vi "FindFirstTouch.vi"(6 "EN":bool, 8 "Level Reference":dbl, 11 "Analog FW In":T1) -> (1 "CounterDeleteOut":i32, 2 "TotalSizeOut":i32, 3 "Analog FW Out":T1)   [LabVIEW 2017]
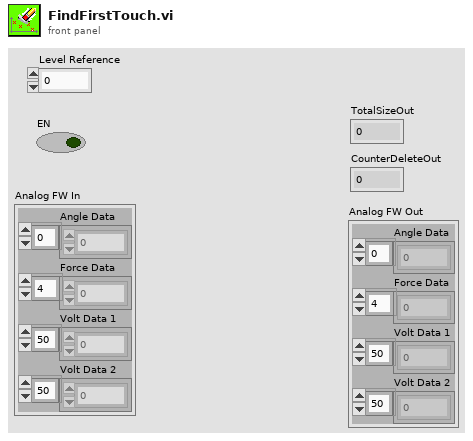
[diagram p1: front panel]
types:
  T1 = cluster{"Angle Data":dbl[], "Force Data":dbl[], "Volt Data 1":dbl[], "Volt Data 2":dbl[]}
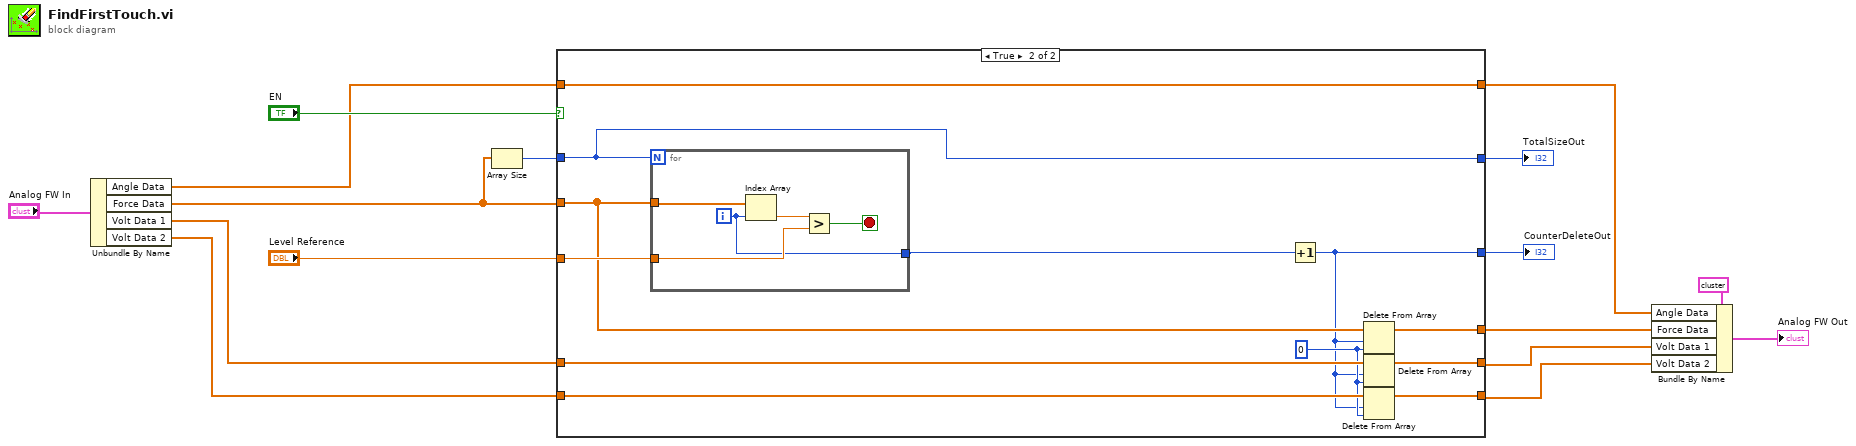
[diagram p0: block diagram]
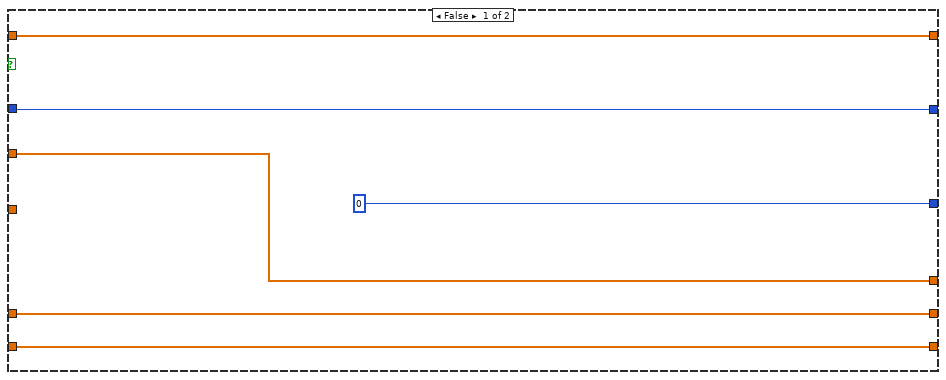
[diagram p2: hidden frame]
diagram:
  n1 = Unbundle By Name("Analog FW In") -> ("Angle Data"=w1:dbl[], "Force Data"=w5:dbl[], "Volt Data 1"=w10:dbl[], "Volt Data 2"=w9:dbl[])
  n2 = Array Size(array=w5) -> (size(s)=w4:i32)
  n3 = case shown="True" "EN" {
    tunnel: "Level Reference" -> [_ w34]
    tunnel: w5 -> [w22 w33]
    tunnel: [w22 w32] -> w11
    tunnel: w10 -> [w21 w31]
    tunnel: w9 -> [w20 w30]
    tunnel: [w21 w28] -> w8
    tunnel: [w20 w27] -> w7
    tunnel: [0 w26] -> w6
    tunnel: w4 -> [w19 w25]
    tunnel: [w19 w25] -> w3
    tunnel: [w17 w24] -> w2
    tunnel: w1 -> [w17 w24]
    frame False {
    }
    frame True {
      w29 = 0 ("index")
      n4 = for {
        N: w25 -> [_]
        tunnel: w33 -> [w39]
        tunnel: w34 -> [w37]
        tunnel: [w35] -> w23
        i -> [w35]
        stop <- w36 stop-if-true
        n5 = Index Array(array=w39, index=w35) -> (element=w38:dbl)
        n6 = Greater?(x=w38, y=w37) -> (0:w36:bool)
      }
      n7 = Increment(x=w23) -> (x+1=w26:i32)
      n8 = Delete From Array "Delete From Array"(array=w33, length=w26, index=w29) -> (array with subset deleted=w32:dbl[])  [unwired: 1 out]
      n9 = Delete From Array(array=w31, length=w26, index=w29) -> (array with subset deleted=w28:dbl[])  [unwired: 1 out]
      n10 = Delete From Array(array=w30, length=w26, index=w29) -> (array with subset deleted=w27:dbl[])  [unwired: 1 out]
    }
  }
  "CounterDeleteOut" <- w6
  "TotalSizeOut" <- w3
  n11 = Bundle By Name(cluster=T1 {"Angle Data"=[], "Force Data"=[0.0, 0.035, 0.005, 0.035, 0.035, 0.035, 0.035, 0.005, 0.005, 0.035, 0.035, 0.035, 0.035, 0.005, 0.065, 0.035, 0.005, 0.035, 0.005, 0.005, 0.005, 0.005, 0.065, 0.035, 0.035, 0.005, 0.035, 0.035, 0.035, 0.065, 0.035, 0.065, 0.035, 0.035, 0.035, 0.035, 0.005, 0.065, 0.035, 0.005, 0.035, 0.035, 0.005, 0.005, 0.035, 0.035, 0.005, 0.065, 0.005, 0.035, 0.026, 0.035, 0.005, 0.035, 0.065, 0.035, 0.035, 0.005, 0.005, 0.035, 0.035, 0.005, 0.005, 0.065, 0.035, 0.035, 0.035, 0.005, 0.065, 0.005, 0.035, 0.005, 0.065, 0.096, 0.065, 0.065, 0.096, 0.035, 0.065, 0.065, 0.096, 0.096, 0.096, 0.096, 0.126, 0.096, 0.096, 0.126, 0.096, 0.126, 0.126, 0.096, 0.218, 0.157, 0.157, 0.187, 0.157, 0.157, 0.187, 0.157, 0.187, 0.218, 0.187, 0.187, 0.187, 0.218, 0.218, 0.248, 0.279, 0.279, 0.279, 0.34, 0.279, 0.279, 0.279, 0.309, 0.279, 0.279, 0.309, 0.34, 0.37, 0.309, 0.37, 0.34, 0.34, 0.401, 0.401, 0.37, 0.401, 0.401, 0.401, 0.37, 0.431, 0.431, 0.431, 0.431, 0.401, 0.462, 0.401, 0.431, 0.431, 0.431, 0.462, 0.431, 0.431, 0.431, 0.431, 0.462, 0.431, 0.431, 0.462, 0.431, 0.431, 0.431, 0.462, 0.431, 0.431, 0.462, 0.401, 0.462, 0.431, 0.431, 0.431, 0.431, 0.462, 0.462, 0.431, 0.462, 0.431, 0.492, 0.431, 0.462, 0.492, 0.431, 0.492, 0.492, 0.492, 0.431, 0.431, 0.522, 0.492, 0.431, 0.462, 0.462, 0.462, 0.492, 0.431, 0.431, 0.431, 0.431, 0.462, 0.462, 0.462, 0.462, 0.401, 0.492, 0.431, 0.431, 0.431, 0.431, 0.431, 0.431, 0.431, 0.431, 0.462, 0.401, 0.431, 0.431, 0.431, 0.431, 0.401, 0.431, 0.431, 0.431, 0.37, 0.431, 0.401, 0.431, 0.401, 0.431, 0.401, 0.431, 0.431, 0.522, 0.462, 0.492, 0.492, 0.522, 0.462, 0.522, 0.522, 0.553, 0.553, 0.553, 0.583, 0.553, 0.583, 0.553, 0.553, 0.553, 0.583, 0.583, 0.614, 0.644, 0.614, 0.614, 0.644, 0.644, 0.644, 0.675, 0.644, 0.675, 0.644, 0.675, 0.705, 0.644, 0.705, 0.766, 0.736, 0.736, 0.766, 0.736, 0.766, 0.766, 0.736, 0.797, 0.766, 0.797, 0.797, 0.766, 0.766, 0.766, 0.797, 0.766, 0.827, 0.827, 0.827, 0.797, 0.827, 0.827, 0.858, 0.858, 0.827, 0.827, 0.766, 0.675, 0.583, 0.492, 0.492, 0.492, 0.492, 0.492, 0.492, 0.492, 0.492, 0.431, 0.462, 0.401, 0.462, 0.462, 0.431, 0.462, 0.462, 0.431, 0.462, 0.462, 0.431, 0.462, 0.462, 0.431, 0.431, 0.462, 0.401, 0.401, 0.431, 0.431, 0.431, 0.431, 0.431, 0.401, 0.431, 0.431, 0.401, 0.431, 0.431, 0.431, 0.431, 0.431, 0.431, 0.431, 0.462, 0.431, 0.462, 0.431, 0.401, 0.431, 0.462, 0.431, 0.492, 0.431, 0.522, 0.553, 0.614, 0.644, 0.644, 0.705, 0.736, 0.797, 0.827, 0.858, 0.888, 0.919, 0.919, 0.949, 1.01, 1.01, 1.04, 1.04, 1.132, 1.101, 1.132, 1.132, 1.162, 1.193, 1.223, 1.254, 1.254, 1.284, 1.315, 1.315, 1.376, 1.436, 1.376, 1.467, 1.467, 1.497, 1.497, 1.589, 1.558, 1.589, 1.619, 1.65, 1.68, 1.741, 1.711, 1.802, 1.802, 1.833, 1.863, 1.893, 1.924, 1.954, 1.985, 1.954, 1.954, 1.954, 1.954, 1.924, 1.924, 1.924, 1.954, 1.924, 1.924, 1.893, 1.954, 1.863, 1.893, 1.893, 1.863, 1.893, 1.893, 1.893, 1.893, 1.893, 1.924, 1.893, 1.924, 1.863, 1.863, 1.863, 1.893, 1.893, 1.863, 1.863, 1.893, 1.863, 1.863, 1.863, 1.893, 1.893, 1.833, 1.893, 1.863, 1.863, 1.802, 1.863, 1.833, 1.863, 1.863], "Volt Data 1"=array[439 elements], "Volt Data 2"=[0.0, 0.036, 0.036, 0.066, 0.005, 0.025, 0.036, 0.036, 0.025, 0.117, 0.036, 0.025, 0.056, 0.066, 0.056, 0.086, 0.036, 0.005, 0.025, 0.036, 0.066, 0.056, 0.086, 0.066, 0.066, 0.036, 0.005, 0.066, 0.036, 0.005, 0.066, 0.036, 0.066, 0.025, 0.005, 0.066, 0.036, 0.056, 0.005, 0.086, 0.025, 0.086, 0.178, 0.036, 0.025, 0.066, 0.056, 0.066, 0.036, 0.025, 0.025, 0.025, 0.066, 0.005, 0.036, 0.066, 0.147, 0.025, 0.025, 0.005, 0.127, 0.086, 0.086, 0.005, 0.005, 0.097, 0.036, 0.005, 0.025, 0.025, 0.086, 0.025, 0.025, 0.066, 0.066, 0.036, 0.056, 0.127, 0.056, 0.056, 0.005, 0.036, 0.005, 0.066, 0.127, 0.056, 0.005, 0.036, 0.005, 0.005, 0.066, 0.056, 0.005, 0.117, 0.036, 0.005, 0.219, 0.056, 0.056, 0.025, 0.005, 0.005, 0.025, 0.056, 0.005, 0.066, 0.025, 0.056, 0.086, 0.025, 0.005, 0.097, 0.025, 0.025, 0.097, 0.097, 0.066, 0.056, 0.066, 0.127, 0.066, 0.097, 0.036, 0.066, 0.005, 0.036, 0.086, 0.066, 0.066, 0.097, 0.036, 0.005, 0.066, 0.005, 0.056, 0.005, 0.066, 0.005, 0.036, 0.025, 0.066, 0.066, 0.005, 0.036, 0.066, 0.158, 0.056, 0.066, 0.036, 0.056, 0.056, 0.036, 0.036, 0.005, 0.036, 0.005, 0.005, 0.005, 0.036, 0.066, 0.066, 0.025, 0.036, 0.005, 0.036, 0.005, 0.066, 0.097, 0.056, 0.036, 0.005, 0.056, 0.025, 0.036, 0.036, 0.036, 0.005, 0.066, 0.005, 0.005, 0.036, 0.066, 0.025, 0.036, 0.025, 0.036, 0.066, 0.086, 0.097, 0.025, 0.056, 0.025, 0.036, 0.025, 0.005, 0.117, 0.086, 0.025, 0.005, 0.066, 0.036, 0.066, 0.005, 0.005, 0.005, 0.066, 0.025, 0.066, 0.056, 0.066, 0.036, 0.036, 0.005, 0.005, 0.025, 0.086, 0.005, 0.066, 0.158, 0.025, 0.127, 0.025, 0.036, 0.005, 0.066, 0.025, 0.036, 0.066, 0.005, 0.086, 0.025, 0.005, 0.066, 0.097, 0.025, 0.005, 0.025, 0.066, 0.127, 0.066, 0.036, 0.005, 0.066, 0.005, 0.025, 0.036, 0.056, 0.066, 0.025, 0.036, 0.036, 0.025, 0.005, 0.025, 0.086, 0.056, 0.127, 0.005, 0.036, 0.025, 0.005, 0.025, 0.066, 0.005, 0.025, 0.036, 0.005, 0.086, 0.066, 0.036, 0.025, 0.117, 0.066, 0.066, 0.066, 0.025, 0.086, 0.025, 0.036, 0.036, 0.036, 0.066, 0.036, 0.066, 0.097, 0.066, 0.097, 0.086, 12.05, 12.111, 12.019, 12.08, 12.08, 12.08, 12.05, 12.019, 12.08, 12.05, 12.019, 12.111, 12.08, 12.05, 12.019, 12.141, 12.08, 12.08, 12.019, 12.08, 12.05, 12.111, 12.019, 12.05, 12.111, 12.08, 12.019, 12.08, 12.05, 12.08, 12.019, 12.08, 12.019, 12.08, 12.019, 12.08, 12.019, 12.05, 12.08, 12.05, 12.111, 12.111, 12.05, 12.05, 12.08, 12.05, 12.08, 12.05, 12.05, 12.05, 12.05, 12.05, 12.111, 12.08, 12.08, 12.111, 12.08, 11.958, 12.019, 12.019, 12.05, 12.08, 12.111, 12.05, 12.08, 12.08, 11.989, 12.05, 12.019, 12.08, 12.111, 12.019, 12.08, 11.989, 12.019, 11.867, 12.019, 12.111, 12.05, 12.08, 12.08, 12.08, 12.019, 12.08, 12.08, 12.08, 12.05, 12.05, 12.05, 12.08, 12.019, 12.019, 12.019, 12.019, 12.05, 12.019, 12.019, 12.05, 11.989, 12.111, 12.141, 12.08, 11.958, 12.05, 11.989, 12.08, 11.989, 12.141, 12.019, 12.111, 12.111, 12.05, 12.05, 12.08, 12.05, 12.019, 12.019, 12.08, 11.989, 12.111, 12.141, 12.05, 12.05, 12.08, 12.08, 12.05, 12.08, 12.019, 12.019, 12.05, 12.111, 12.05, 12.08, 12.05, 11.958, 12.08, 12.05, 12.172, 11.989, 12.05, 12.05, 12.08, 12.08, 12.08, 12.05, 12.05, 12.111, 12.08, 12.05, 12.05, 12.141]} ("Analog FW Out"), "Angle Data"=w2, "Force Data"=w11, "Volt Data 1"=w8, "Volt Data 2"=w7) -> (→"Analog FW Out":T1)
